vi "Write Ctls.vi"(10 "控件":T1, 11 "冷却器UI输入":refnum<class "Live User Controller.lvclass">) -> (3 "冷却器UI输出":refnum<class "Live User Controller.lvclass">)   [LabVIEW 2015, in "Live User Controller.lvclass"]
doc: "将用户接口的控件引用句柄写入操作者对象。"
uses:
  Live User Controller.lvclass
  ControlRefs.ctl
  Live User Controller.lvclass/Live User Controller.ctl
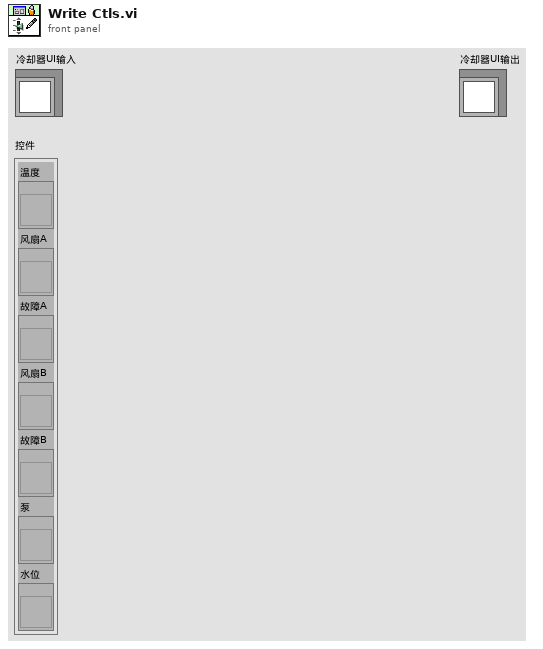
[diagram p1: front panel]
types:
  T1 = typedef "Live User Controller.lvclass/ControlRefs.ctl" = cluster{"温度":refnum<vi>, "风扇A":refnum<vi>, "故障A":refnum<vi>, "风扇B":refnum<vi>, "故障B":refnum<vi>, "泵":refnum<vi>, "水位":refnum<vi>}
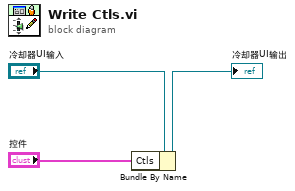
[diagram p0: block diagram]
diagram:
  n1 = Bundle By Name(cluster="冷却器UI输入", "Ctls"="控件") -> (→"冷却器UI输出":refnum<class "Live User Controller.lvclass">)
